vi "CalFile2Info.vi"(0 "Calibration File":path, 1 "Sensors Active":bool[](array[boolean])=[TRUE, TRUE, TRUE, TRUE, TRUE, TRUE, FALSE, FALSE, TRUE, TRUE, FALSE, TRUE, TRUE, TRUE, FALSE, TRUE, TRUE, TRUE, FALSE, TRUE, TRUE, TRUE, TRUE, FALSE]) -> (3 "Calibration Array":cluster{"Offset":dbl, "Gain":dbl}[](array[cluster]))   [LabVIEW 2012]
doc: "This program loads the calibration file generated by either CgCalibrate or the DCU program from the cyberglove. Using the a binary array of sensors active it produces a calibration array of gains and offsets for the sensors that will be outputted from the cyberglove."
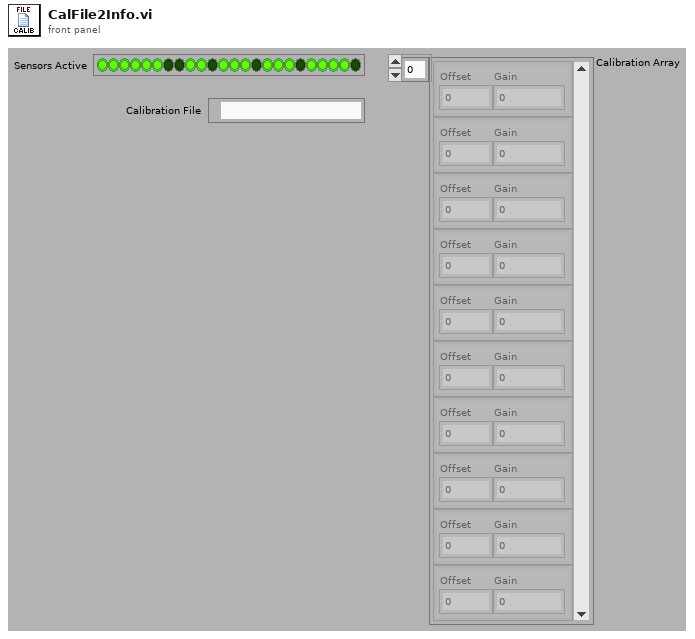
[diagram p1: front panel]
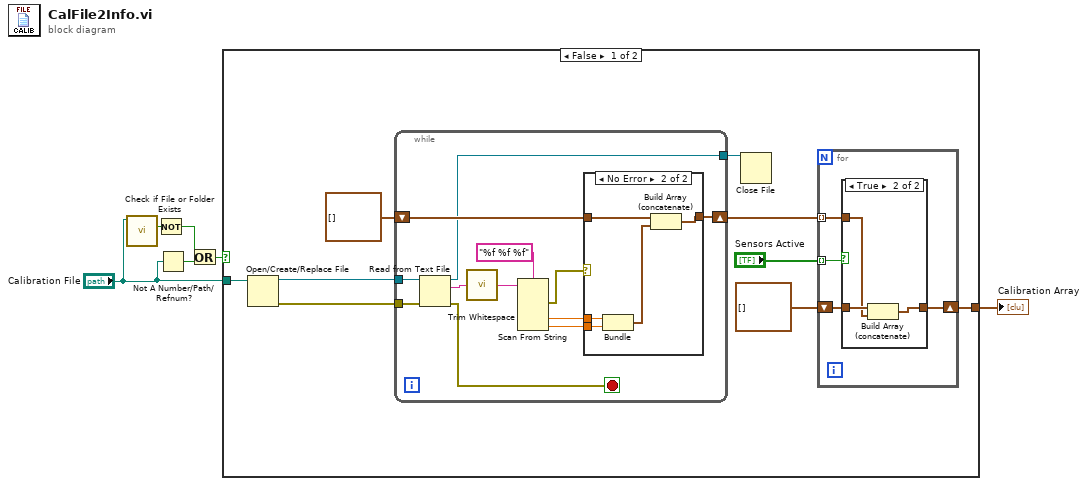
[diagram p0: block diagram]
diagram:
  n1 = call <vilib>:"Check if File or Folder Exists.vi"("path"="Calibration File") -> ("file or folder exists?"=w4:bool)  [unwired: 8 in, 2 out]
  n2 = Not(x=w4) -> (.not. x?=w2:bool)
  n3 = Not A Number/Path/Refnum?(number/path/refnum="Calibration File") -> (NaN/Path/Refnum?=w3:bool)
  n4 = Or(x=w2, y=w3) -> (x .or. y?=w1:bool)
  n5 = case shown="False" w1 {
    tunnel: [w10 _] -> w6
    tunnel: "Calibration File" -> [w8 _]
    frame False {
      n6 = Open/Create/Replace File(file path (use dialog)=w8) -> (refnum out=w15:refnum<file>, error out=w7:errorcluster)  [unwired: 5 in, 1 out]
      n7 = while {
        tunnel: w15 -> [w35]
        shift-right: [w29] -> w13
        shift-left: cluster{dbl, dbl}[] [] -> [w28]
        tunnel: [w25] -> w9
        tunnel: w7 -> [w24]
        stop <- w26 stop-if-true
        n8 = Read from Text File(file (use dialog)=w35, error in=w24) -> (refnum out=w25:refnum<file>, text=w34:string, error out=w26:errorcluster)  [unwired: 2 in, 1 out]
        n9 = call <vilib>:"Trim Whitespace.vi"("string"=w34) -> ("trimmed string"=w33:string)  [unwired: 1 in]
        n10 = Scan From String(format string="%f %f %f", input string=w33) -> (error out=w27:errorcluster, output 2=w31:dbl, output 3=w30:dbl)  [unwired: 6 in, 2 out]
        n11 = case shown="No Error" w27 {
          tunnel: w31 -> [_ w41]
          tunnel: w30 -> [_ w40]
          tunnel: [w36 w38] -> w29
          tunnel: w28 -> [w36 w37]
          frame Error {
          }
          frame No Error {
            n12 = Bundle(w41, w40) -> (w39:cluster{dbl, dbl})  [unwired: 1 in]
            n13 = Build Array (concatenate)(w37, w39) -> (w38:cluster{dbl, dbl}[])
          }
        }
      }
      n14 = Close File(refnum=w9) -> ()  [unwired: 1 in, 2 out]
      n15 = for {
        tunnel: w13 -> [w18] mode=indexing
        tunnel: "Sensors Active" -> [w19] mode=indexing
        shift-right: [w16] -> w10
        shift-left: cluster{"Offset":dbl, "Gain":dbl}[] [] ("Array") -> [w17]
        n16 = case shown="True" w19 {
          tunnel: w18 -> [_ w21]
          tunnel: w17 -> [w20 w22]
          tunnel: [w20 w23] -> w16
          frame False {
          }
          frame True {
            n17 = Build Array (concatenate)(w22, w21) -> (w23:cluster{"Offset":dbl, "Gain":dbl}[])
          }
        }
      }
    }
    frame True {
    }
  }
  "Calibration Array" <- w6
